vi "C37 Read SGL Array from Pointer.vi"(9 "Array Length":i32, 10 "Pointer":u32, 11 "Data is Valid":bool) -> (3 "Values":sgl[](array[numeric]))   [LabVIEW 2018, in "S3DK.lvlib" / "C37118-DLL.lvlib"]
uses:
  C37118-DLL.lvlib
  <vilib>/Utility/importsl/GetValueByPointer/datatype.ctl
  <vilib>/Utility/importsl/GetValueByPointer/GetValueByPointer.xnode
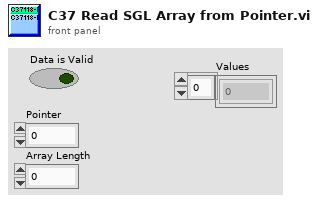
[diagram p1: front panel]
types:
  T1 = enum32{"pack1", "pack2", "pack4", "pack8", "pack16"}
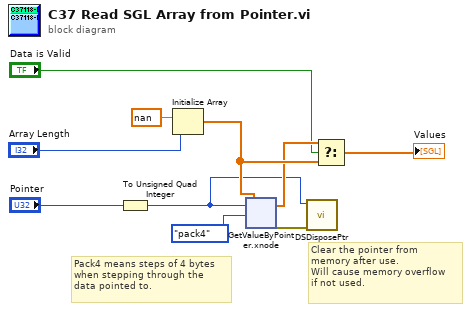
[diagram p0: block diagram]
diagram:
  # "Clear the pointer from \nmemory after use.\nWill cause memory overflow\nif not used."
  # "Pack4 means steps of 4 bytes \nwhen stepping through the \ndata pointed to."
  n1 = To Unsigned Quad Integer(1:"Pointer") -> (0:w8:u64)
  n2 = Initialize Array(sgl nan ("phasorValueReal"), "Array Length") -> (w10:sgl[])
  n3 = xnode "GetValueByPointer.xnode"("Pointer"=w8, "InputType"=w10, "PackType"=T1."pack4") -> ("Output"=w9:sgl[], "ErrorOut"=w6:errorcluster)  [unwired: 1 in]
  n4 = call <vilib>:"DSDisposePtr.vi"("error in (no error)"=w6, "Pointer"=w8) -> ()  [unwired: 9 in, 1 out]
  n5 = Select(t=w9, s="Data is Valid", f=w10) -> (s? t:f=→"Values":sgl[])
